vi "Start_Balancing.vi"(8 "error in":errorcluster, 9 "Hz":dbl) -> (0 "error out":errorcluster)   [LabVIEW 2014]
uses:
  Start.vi
  Saturation_Counter.vi
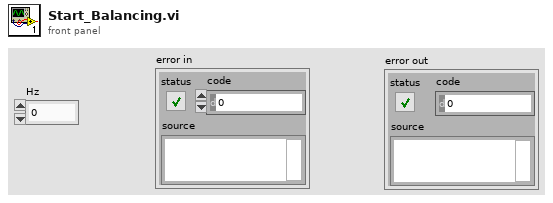
[diagram p1: front panel]
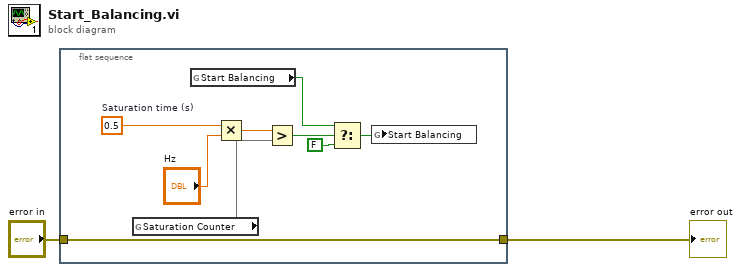
[diagram p0: block diagram]
diagram:
  n1 = flat-sequence {
    tunnel: [w3] -> w1
    tunnel: "error in" -> [w3]
    frame #0 {
      w7 = 0.5  # Saturation time (s)
      n2 = global read "Saturation_Counter.vi" "Saturation Counter"() -> (w10)
      n3 = global read "Start.vi" "Start Balancing"() -> (w4:bool)
      n4 = Multiply(x=w7, y="Hz") -> (x*y=w9:dbl)
      n5 = Greater?(x=w9, y=w10) -> (0:w5:bool)
      n6 = Select(t=w4, s=w5, f=FALSE) -> (s? t:f=w6:bool)
      n7 = global write "Start.vi" "Start Balancing"(w6) -> ()
    }
  }
  "error out" <- w1
